vi "DAQ_AO.vi"(8 "error in":errorcluster, 10 "Operatin":enum16{"Set", "Initialize"}(ring)) -> (0 "error out":errorcluster, 3 "SettingData":dbl[](array[numeric]) format="%0.2f")   [LabVIEW 2013]
uses:
  <vilib>/DAQmx/write.llb/DAQmx Write (Analog DBL 1Chan 1Samp).vi
  <vilib>/DAQmx/create/channels.llb/DAQmx Create Channel (AO-Voltage-Basic).vi
  <vilib>/DAQmx/miscellaneous.llb/DAQmx Fill In Error Info.vi
panel:
  in  "data":dbl[](array[numeric]) caption="数据" format="%0.2f"
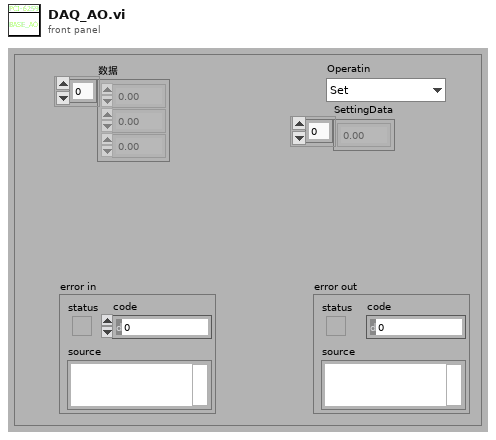
[diagram p1: front panel]
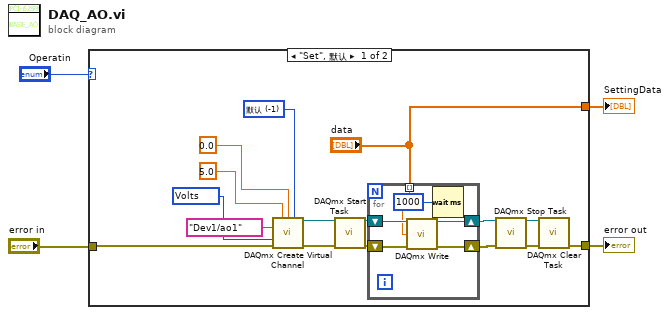
[diagram p0: block diagram]
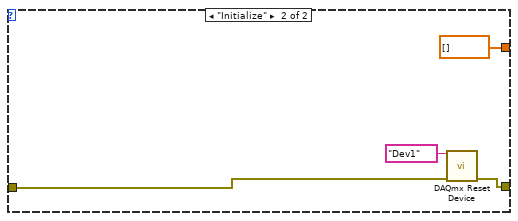
[diagram p2: hidden frame]
diagram:
  n1 = case shown="\"Set\", 默认" "Operatin" {
    tunnel: "error in" -> [w7 w30]
    tunnel: [w16 w29] -> w3
    tunnel: ["data" dbl[] [] ("data 2")] -> w1
    frame "Set", Default {
      w5 = -1 items=["默认"=-1, "RSE"=10083, "差分"=10106, "伪差分"=12529] ("output terminal configuration")
      w13 = 10348 items=["Volts"=10348, "From Custom Scale"=10065] ("units")
      n2 = call-poly <vilib>:"DAQmx Create Virtual Channel.vi"("maximum value"=5.0, "minimum value"=0.0, "output terminal configuration"=w5, "physical channels"=tag "Dev1/ao1", "units"=w13, "error in"=w7) -> ("task out"=w9:refnum<k21>, "error out"=w10:errorcluster)  [unwired: 8 in]
      n3 = call <vilib>:"DAQmx Start Task.vi"("task/channels in"=w9, "error in"=w10) -> ("task out"=w20:refnum<k21>, "error out"=w19:errorcluster)  [unwired: 12 in]
      n4 = for {
        tunnel: "data" -> [w22] mode=indexing
        shift-right: [w24] -> w15
        shift-left: w20 -> [w26]
        shift-right: [w23] -> w14
        shift-left: w19 -> [w25]
        n5 = call-poly <vilib>:"DAQmx Write.vi"("task/channels in"=w26, "data"=w22, "error in"=w25) -> ("task out"=w24:refnum<k21>, "error out"=w23:errorcluster)  [unwired: 10 in, 1 out]
        n6 = Wait (ms)(milliseconds to wait=u32 1000 ("等待时间（毫秒）")) -> ()  [unwired: 1 out]
      }
      n7 = call <vilib>:"DAQmx Stop Task.vi"("task/channels in"=w15, "error in"=w14) -> ("task out"=w18:refnum<k21>, "error out"=w17:errorcluster)  [unwired: 12 in]
      n8 = call <vilib>:"DAQmx Clear Task.vi"("task in"=w18, "error in"=w17) -> ("error out"=w16:errorcluster)  [unwired: 13 in]
    }
    frame "Initialize" {
      n9 = call <vilib>:"DAQmx Reset Device.vi"("device in"=tag "Dev1", "error in"=w30) -> ("error out"=w29:errorcluster)  [unwired: 13 in]
    }
  }
  "error out" <- w3
  "SettingData" <- w1
